vi "Convert Detection Robot to AI Robot.vi"(7 "Lado":enum16{"Esquerdo", "Direito"}(ring) caption="Enum", 11 "Input":T4[](array[typedef]) {"orientation" format="%+4.3f"; "y" format="%+4.3f"; "confidence" format="%4.3f"; "x" format="%+4.3f"}) -> (3 "Output":T1[](array[typedef]))   [LabVIEW 2017]
uses:
  SSL Detection Robot.ctl
  <vilib>/Analysis/Matrix/Datatypes/RealMatrix.ctl
  AI Robot.ctl
  Intel/Functions Enum.ctl
  Intel/AttackerStates.ctl
  <vilib>/Analysis/Matrix/NI_Matrix.lvlib
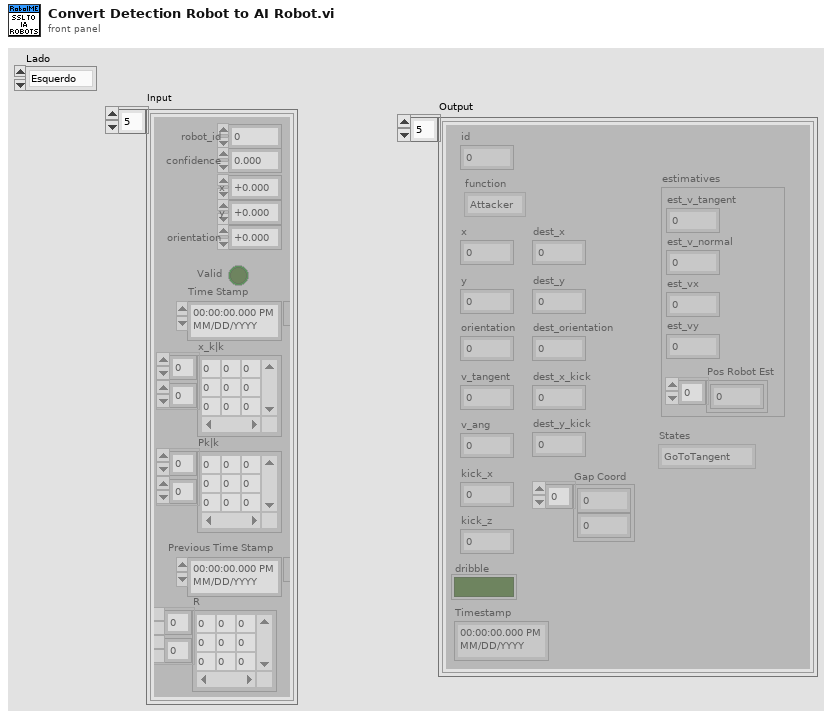
[diagram p1: front panel]
types:
  T1 = typedef "AI Robot.ctl" = cluster{"id":u32, "function":T2, "x":dbl, "y":dbl, "orientation":dbl, "v_tangent":dbl, "v_ang":dbl, "kick_x":dbl, "kick_z":dbl, "dribble":bool, "Timestamp":timestamp, "dest_x":dbl, "dest_y":dbl, "dest_orientation":dbl, "estimatives":cluster{"est_v_tangent":dbl, "est_v_normal":dbl, "est_vx":dbl, "est_vy":dbl, "Pos Robot Est":dbl[]}, "dest_x_kick":dbl, "dest_y_kick":dbl, "Gap Coord":dbl[], "States":T3}
  T2 = typedef "Functions Enum.ctl" = enum16{"Attacker", "Goalie", "Defender", "Striker", "Goto 0", "Dummy", "Kicker", "ZigZag"}
  T3 = typedef "AttackerStates.ctl" = enum16{"Pass", "GoToTangent", "BallGetting", "GoToKick", ""}
  T4 = typedef "SSL Detection Robot.ctl" = cluster{"x":sgl, "robot_id":u32, "confidence":sgl, "y":sgl, "orientation":sgl, "Valid":bool, "Time Stamp":timestamp, "x_k|k":T5, "Pk|k":T5, "Previous Time Stamp":timestamp, "R":T5}
  T5 = typedef "NI_Matrix.lvlib/RealMatrix.ctl" = dbl[][]
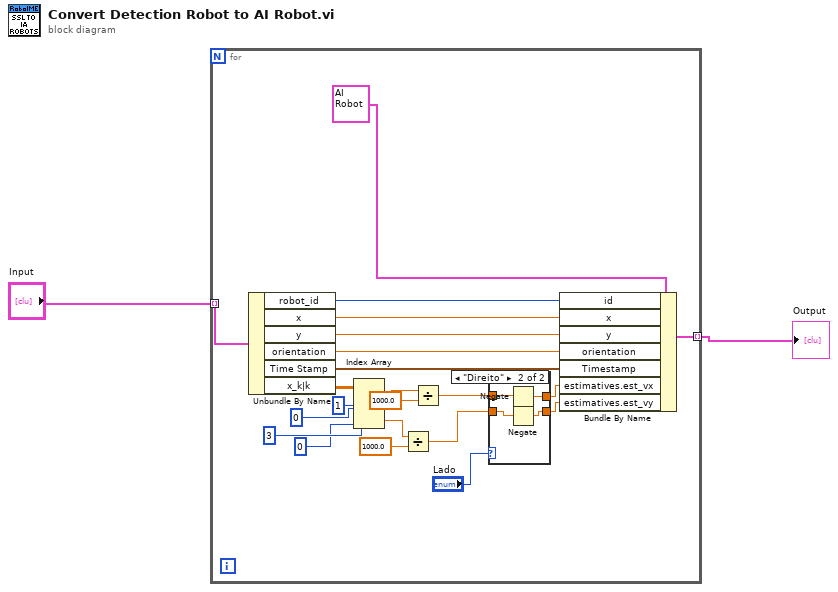
[diagram p0: block diagram]
diagram:
  n1 = for {
    tunnel: "Input" -> [w23] mode=indexing
    tunnel: [w17] -> w1 mode=indexing
    n2 = Unbundle By Name(w23) -> ("robot_id"=w22:u32, "x"=w21:sgl, "y"=w20:sgl, "orientation"=w19:sgl, "Time Stamp"=w18:timestamp, "x_k|k"=w16:T5)
    n3 = Index Array(array=w16, index (row) #1=1 ("index (row)"), index (col) #1=0 ("disabled index (col)"), index (row) #2=3 ("index (row)"), index (col) #2=0 ("disabled index (col)")) -> (element #1=w11:dbl, element #2=w8:dbl)
    n4 = Divide(x=w8, y=1000.0) -> (x/y=w4:dbl)
    n5 = Divide(x=w11, y=1000.0) -> (x/y=w6:dbl)
    n6 = case shown="\"Direito\"" "Lado" {
      tunnel: [w26 w30] -> w5
      tunnel: w6 -> [w26 w29]
      tunnel: [w25 w27] -> w3
      tunnel: w4 -> [w25 w28]
      frame "Esquerdo", Default {
      }
      frame "Direito" {
        n7 = Negate(x=w29) -> (-x=w30:dbl)
        n8 = Negate(x=w28) -> (-x=w27:dbl)
      }
    }
    n9 = Bundle By Name(cluster=T1 {"id"=0, "function"=enum."Attacker", "x"=0.0, "y"=0.0, "orientation"=0.0, "v_tangent"=0.0, "v_ang"=0.0, "kick_x"=0.0, "kick_z"=0.0, "dribble"=FALSE, "Timestamp"=timestamp(0 s since 1904-01-01), "dest_x"=0.0, "dest_y"=0.0, "dest_orientation"=0.0, "estimatives"={"est_v_tangent"=0.0, "est_v_normal"=0.0, "est_vx"=0.0, "est_vy"=0.0, "Pos Robot Est"=[]}, "dest_x_kick"=0.0, "dest_y_kick"=0.0, "Gap Coord"=[], "States"=enum."GoToTangent"} ("Robot"), "id"=w22, "x"=w21, "y"=w20, "orientation"=w19, "Timestamp"=w18, "estimatives.est_vx"=w5, "estimatives.est_vy"=w3) -> (w17:T1)
  }
  "Output" <- w1
